vi "setUp.vi"(8 "error in (no error)":errorcluster, 11 "reference in":refnum<class "StringList_Delegations.lvclass">) -> (0 "error out":errorcluster, 3 "reference in":refnum<class "StringList_Delegations.lvclass">)   [LabVIEW 2009, in "StringList_Delegations.lvclass"]
doc: "setUp runs prior to the test method during test execution. Use this method to initialize any object data required by your tests."
uses:
  StringList_Delegations.lvclass
  Test Doubles/ListImp_RefSpy/ListImp_RefSpy.lvclass
  StringList_Delegations.lvclass/StringList_Delegations.ctl
  <vilib>/addons/_JKI Toolkits/VI Tester/TestCase.llb/TestCase.lvclass
  source/Lists.Interfaces/StringList/StringList.lvclass
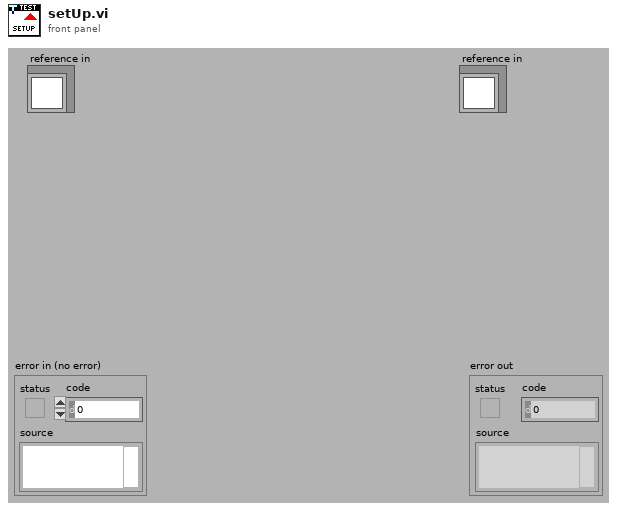
[diagram p1: front panel]
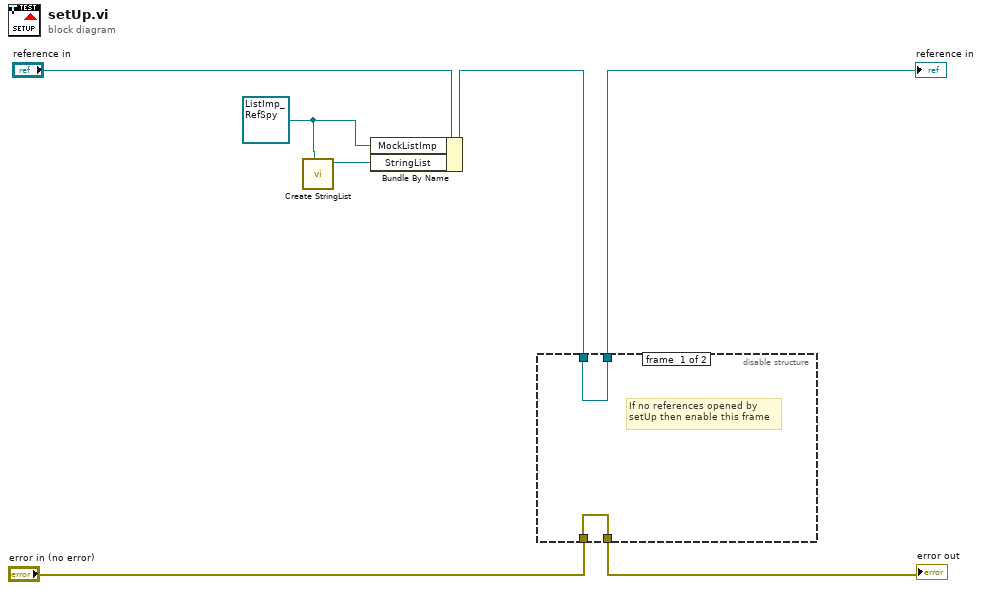
[diagram p0: block diagram]
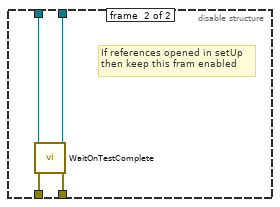
[diagram p2: hidden frame]
diagram:
  w2 = refnum<class "ListImp_RefSpy.lvclass"> refnum ("MockListImp.lvclass")
  n1 = call "Create StringList.vi"("List Implementation (Array)"=w2) -> ("StringList out"=w1:refnum<class "StringList.lvclass">)  [unwired: 9 in, 1 out]
  n2 = Bundle By Name(cluster="reference in", "MockListImp"=w2, "StringList"=w1) -> (w3:refnum<class "StringList_Delegations.lvclass">)
  n3 = disable-structure shown="Enabled" {
    disable-tunnel: w3 -> [w9 w13]
    disable-tunnel: [w9 w12] -> w4
    disable-tunnel: "error in (no error)" -> [w8 w11]
    disable-tunnel: [w8 w10] -> w6
    frame #0 {
      # "If no references opened by\nsetUp then enable this frame"
    }
    frame #1 {
      # "If references opened in setUp\nthen keep this fram enabled"
      n4 = call <vilib>:"WaitOnTestComplete.vi"("error in (no error)"=w11, "TestCase in"=w13) -> ("error out"=w10:errorcluster, "TestCase out"=w12:refnum<class "StringList_Delegations.lvclass">)  [unwired: 8 in]
    }
  }
  "error out" <- w6
  "reference in" <- w4
